vi "Excel_JustCode.vi"(3 "error in (no error)":errorcluster, 4 "JustCode":string[](array[string]), 5 "report in":refnum<class "NI_report.lvclass">) -> (0 "error out":errorcluster, 2 "report out":refnum<class "NI_report.lvclass">)   [LabVIEW 2015]
uses:
  <vilib>/Utility/NIReport.llb/NI_report.lvclass
  CustomControl/TableUnit.ctl
  <vilib>/addons/_office/NI_ReportGenerationToolkit.lvlib
panel:
  in  "start(-1,-1)":T1
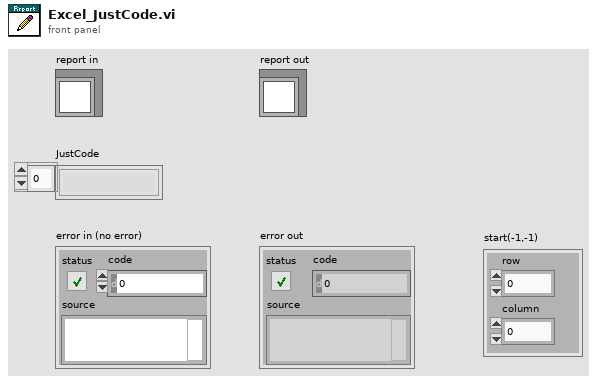
[diagram p1: front panel]
types:
  T1 = typedef "TableUnit.ctl" = cluster{"row":i32, "column":i32}
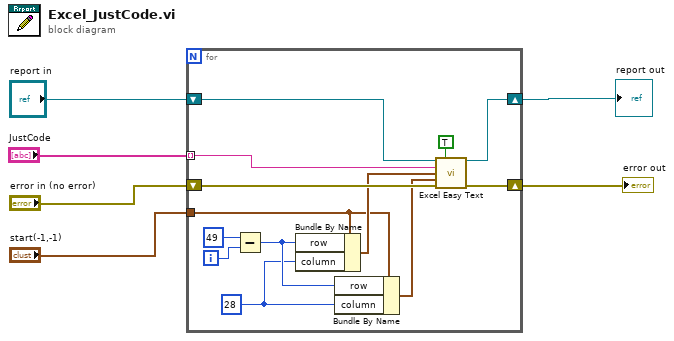
[diagram p0: block diagram]
diagram:
  n1 = for {
    tunnel: "start(-1,-1)" -> [w11]
    shift-right: [w17] -> w2
    shift-left: "error in (no error)" -> [w18]
    shift-right: [w10] -> w3
    shift-left: "report in" -> [w19]
    tunnel: "JustCode" -> [w9] mode=indexing
    i -> [w13]
    w7 = 28 ("column")
    n2 = Subtract(x=49, y=w13) -> (x-y=w14:i32)
    n3 = Bundle By Name(cluster=w11, "row"=w14, "column"=w7) -> (w16:T1)
    n4 = Bundle By Name(cluster=w11, "row"=w14, "column"=w7) -> (w15:T1)
    n5 = call <vilib>:"Excel Easy Text.vi"("report in"=w19, "border? (F)"=TRUE, "text"=w9, "start (-1, -1)"=w16, "end (-1, -1)"=w15, "error in (no error)"=w18) -> ("report out"=w10:refnum<class "NI_report.lvclass">, "error out"=w17:errorcluster)  [unwired: 5 in, 3 out]
  }
  "error out" <- w2
  "report out" <- w3
